vi "Main_Hand_Control_No_Leap_Motion.vi"() -> ()   [LabVIEW 2015]
uses:
  <instrlib>/Dynamixel Motor/Public/Motor Operation/Low Level/Baud Setting.ctl
  <instrlib>/Dynamixel Motor/Dynamixel Motor.lvlib
panel:
  in  "Motors info in":T1(array[cluster])=[{"Motor "="Wrist rotation", "Position (% max position)"=0.0}, {"Motor "="Wrist adduction", "Position (% max position)"=0.0}, {"Motor "="Wrist flexion", "Position (% max position)"=0.0}, {"Motor "="Thumb adduction", "Position (% max position)"=0.0}, {"Motor "="Thumb flexion", "Position (% max position)"=0.0}, {"Motor "="Index flexion", "Position (% max position)"=0.0}, {"Motor "="Middle fingers flexion", "Position (% max position)"=0.0}]
  out "Motors info":T2(array[cluster])
  in  "VISA resource name":refnum<visa-resource-name>="COM9"
  in  "Stop Button":bool
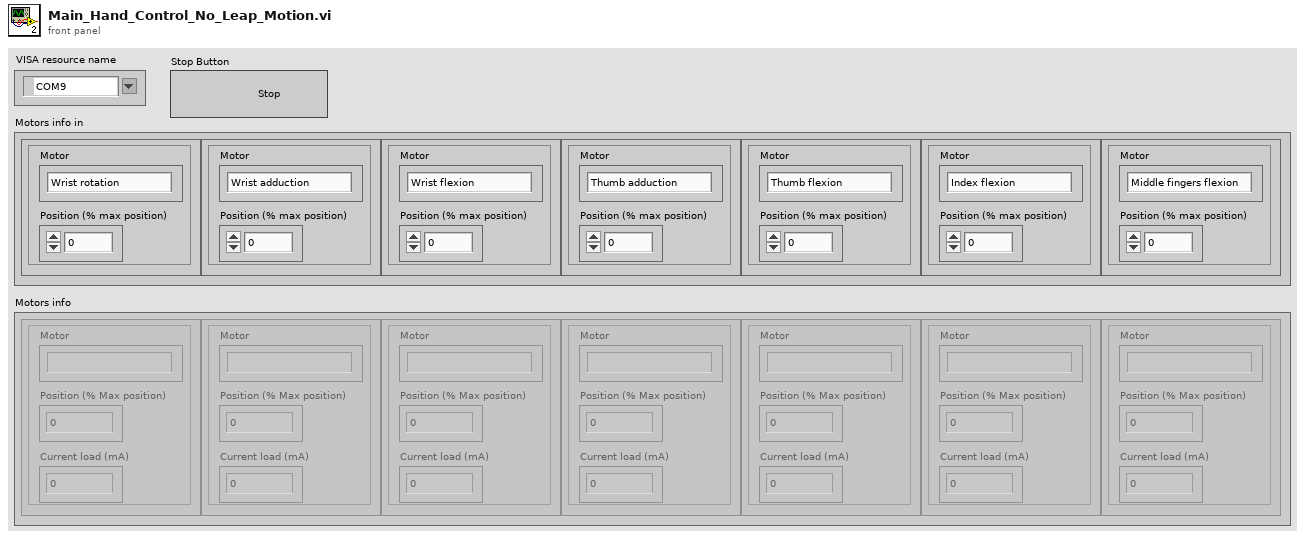
[diagram p1: front panel]
types:
  T1 = cluster{"Motor ":string, "Position (% max position)":dbl}[]
  T2 = cluster{"Motor ":string, "Position (% Max position)":dbl, "Current load (mA)":dbl}[]
  T3 = typedef "Dynamixel Motor.lvlib/Baud Setting.ctl" = u8
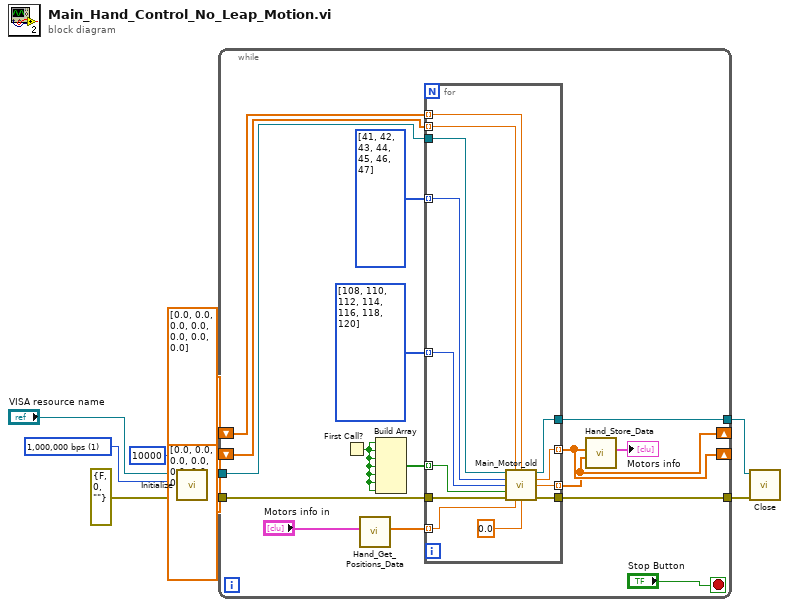
[diagram p0: block diagram]
diagram:
  w10 = T3 1 items=["1,000,000 bps"=1, "500,000 bps"=3, "400,000 bps"=4, "250,000 bps"=7, "200,000 bps"=9, "115200 bps"=16, "57600 bps"=34, "19200 bps"=103, "9600 bps"=207] ("Baud rate (57600 bps)")
  n1 = call <instrlib>:"Initialize.vi"("Timeout (30 msec)"=u32 10000, "error in (no error)"=errorcluster {"status"=FALSE, "code"=0, "source"=""}, "Baud rate (57600 bps)"=w10, "VISA resource name"="VISA resource name") -> ("error out"=w5:errorcluster, "VISA resource name out"=w6:refnum<visa-resource-name>)  [unwired: 6 in]
  n2 = while {
    tunnel: w6 -> [w23]
    tunnel: w5 -> [w22]
    tunnel: [w20] -> w4
    tunnel: [w21] -> w3
    shift-right: [w16] -> _
    shift-left: dbl[] [0.0, 0.0, 0.0, 0.0, 0.0, 0.0, 0.0] -> [w15]
    shift-right: [w14] -> _
    shift-left: dbl[] [0.0, 0.0, 0.0, 0.0, 0.0, 0.0, 0.0] -> [w13]
    stop <- "Stop Button" stop-if-true
    n3 = First Call?() -> (First Call?: T/F=w19:bool)
    n4 = call "Hand_Get_Positions_Data.vi"("Motors info in"="Motors info in") -> ("Positions (bits)"=w17:dbl[])  [unwired: 10 in]
    n5 = Build Array(w19, w19, w19, w19, w19, w19, w19) -> (w18:bool[])
    n6 = for {
      tunnel: w23 -> [w39]
      tunnel: w22 -> [w38]
      tunnel: [w37] -> w21
      tunnel: [w36] -> w20
      tunnel: [w35] -> w16 mode=indexing
      tunnel: [w34] -> w14 mode=indexing
      tunnel: w18 -> [w33] mode=indexing
      tunnel: w17 -> [w32] mode=indexing
      tunnel: w15 -> [w30] mode=indexing
      tunnel: w13 -> [w29] mode=indexing
      tunnel: u8[] [41, 42, 43, 44, 45, 46, 47] ("Motor ID") -> [w28] mode=indexing
      tunnel: u8[] [108, 110, 112, 114, 116, 118, 120] ("Address # DEC") -> [w27] mode=indexing
      n7 = call "Main_Motor_old.vi"("VISA resource name"=w39, "Old Position Motor"=w30, "Old Current load"=w29, "Motor ID"=w28, "Address"=w27, "Torque enable?"=w33, "error in (no error)"=w38, "Goal Position"=w32, "Goal Speed (RPM)"=0.0) -> ("VISA resource name out"=w36:refnum<visa-resource-name>, "New Position Motor"=w35:dbl, "New Current load (mA)"=w34:dbl, "error out"=w37:errorcluster)  [unwired: 3 in]
    }
    n8 = call "Hand_Store_Data.vi"("Current load (mA)"=w14, "Position (bits)"=w16) -> ("Motors info"=→"Motors info":T2)  [unwired: 9 in]
  }
  n9 = call <instrlib>:"Close.vi"("error in (no error)"=w3, "VISA resource name"=w4) -> ()  [unwired: 9 in, 1 out]
